vi "State Tab.vi"(1 "Com Port":T1) -> (0 "Setting Tab":T2(ring)=enum."PLZ Setting")   [LabVIEW 2018]
uses:
  Data Def/Com Port.ctl
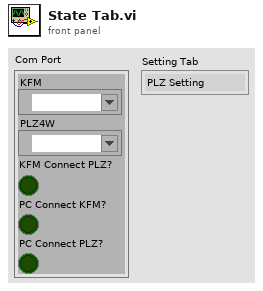
[diagram p1: front panel]
types:
  T1 = typedef "Com Port.ctl" = cluster{"KFM":refnum<visa-resource-name>, "PLZ4W":refnum<visa-resource-name>, "KFM Connect PLZ?":bool, "PC Connect KFM?":bool, "PC Connect PLZ?":bool}
  T2 = enum32{"KFM Setting", "PLZ Setting", "Discoonect"}
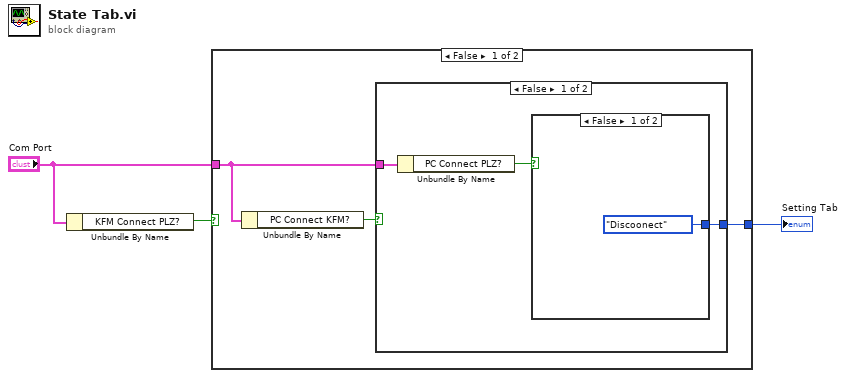
[diagram p0: block diagram]
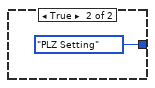
[diagram p2: hidden frame]
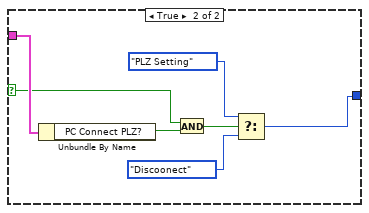
[diagram p3: hidden frame]
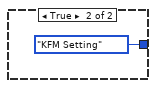
[diagram p4: hidden frame]
diagram:
  n1 = Unbundle By Name("Com Port") -> ("KFM Connect PLZ?"=w3:bool)
  n2 = case shown="False" w3 {
    tunnel: "Com Port" -> [w4 _]
    tunnel: [w5 T2."KFM Setting" ("Setting Tab")] -> w1
    frame False {
      n3 = Unbundle By Name(w4) -> ("PC Connect KFM?"=w6:bool)
      n4 = case shown="False" w6 {
        selector: w6 -> [_ w16]
        tunnel: [w7 w12] -> w5
        tunnel: w4 -> [w8 w18]
        frame False {
          n5 = Unbundle By Name(w8) -> ("PC Connect PLZ?"=w9:bool)
          n6 = case shown="False" w9 {
            tunnel: [T2."Discoonect" ("Setting Tab") T2."PLZ Setting" ("Setting Tab")] -> w7
            frame False {
            }
            frame True {
            }
          }
        }
        frame True {
          n7 = Unbundle By Name(w18) -> ("PC Connect PLZ?"=w17:bool)
          n8 = And(x=w16, y=w17) -> (x .and. y?=w15:bool)
          n9 = Select(t=T2."PLZ Setting" ("Setting Tab"), s=w15, f=T2."Discoonect" ("Setting Tab")) -> (s? t:f=w12:T2)
        }
      }
    }
    frame True {
    }
  }
  "Setting Tab" <- w1
